vi "sensor cmd time get.vi"(0 "device_handle":u32, 1 "year":u32, 2 "month":u32, 3 "day":u32, 4 "hour":u32, 5 "minute":u32, 6 "second":u32) -> (18 "function return":i32, 20 "device_handle out":u32, 21 "year out":u32, 22 "month out":u32, 23 "day out":u32, 24 "hour out":u32, 25 "minute out":u32, 26 "second out":u32)   [LabVIEW 2019, in "apdm.lvlib"]
doc: "APDM_EXPORT int apdm_sensor_cmd_time_get(apdm_device_handle_t device_handle, uint32_t *year, uint32_t *month, uint32_t *day, uint32_t *hour, uint32_t *minute, uint32_t *second);"
uses:
  apdm.lvlib
  Lee Lab/CP FES Walking 2018/Code/Working/LabVIEW/apdm.dll
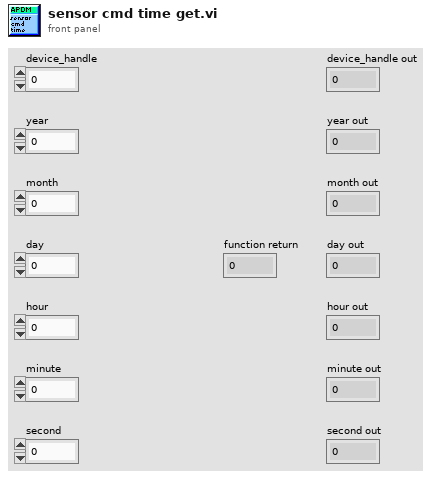
[diagram p1: front panel]
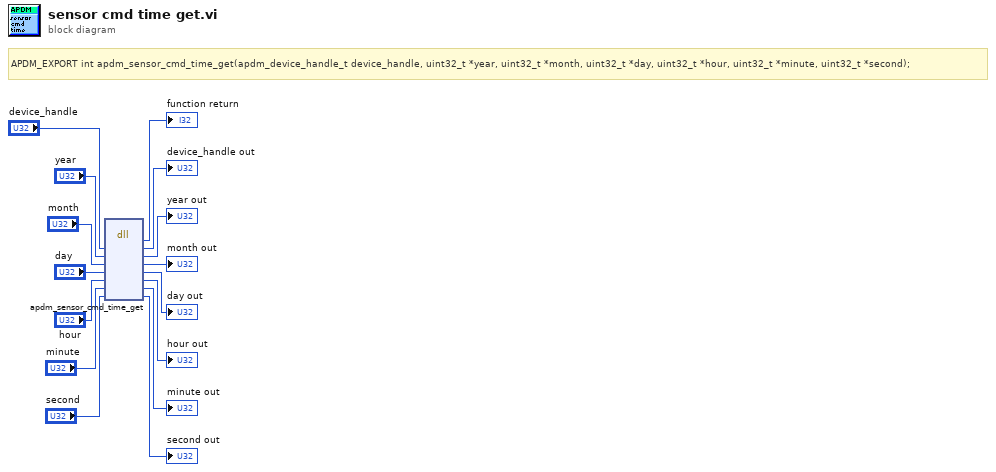
[diagram p0: block diagram]
diagram:
  # "APDM_EXPORT int apdm_sensor_cmd_time_get(apdm_device_handle_t device_handle, uint32_t *year, uint32_t *month, uint32_t *day, uint32_t *hour, uint32_t *minute, uint32_t *second);"
  n1 = dll-call lib="C:/Users/jfalesi/Dropbox/Lee Lab/CP FES Walking 2018/Code/Working/LabVIEW/apdm.*" fn="apdm_sensor_cmd_time_get"("device_handle"="device_handle", "year"="year", "month"="month", "day"="day", "hour"="hour", "minute"="minute", "second"="second") -> (→"function return":i32, "device_handle"=→"device_handle out":u32, "year"=→"year out":u32, "month"=→"month out":u32, "day"=→"day out":u32, "hour"=→"hour out":u32, "minute"=→"minute out":u32, "second"=→"second out":u32)  [unwired: 3 in, 2 out]
